vi "Test Sound Measurement.vi"() -> ()   [LabVIEW 2013]
doc: "This VI is used for testing dynamic pressure measurement acquisition with our dynamic pressure sensors and analog input card."
uses:
  <vilib>/DAQmx/read.llb/DAQmx Read (Analog 1D Wfm NChan NSamp).vi
  <vilib>/measure/maspectr.llb/FFT Power Spectrum and PSD for N Chan.vi
  <vilib>/DAQmx/miscellaneous.llb/DAQmx Fill In Error Info.vi
  <vilib>/measure/NI_MAPro.lvlib
panel:
  out "Dynamic Pressure":cluster{"f0":dbl, "df":dbl, "magnitude":dbl[]}[](graph)
  in  "Stop Button":bool
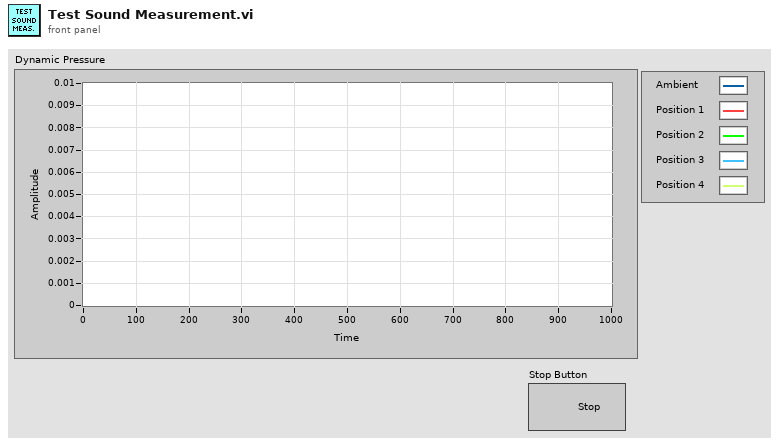
[diagram p1: front panel]
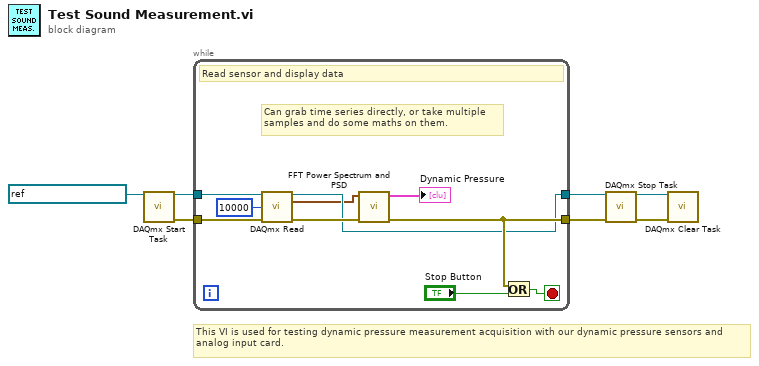
[diagram p0: block diagram]
diagram:
  # "This VI is used for testing dynamic pressure measurement acquisition with our dynamic pressure sensors and analog input card."
  n1 = call <vilib>:"DAQmx Start Task.vi"("task/channels in"=refnum<k21> "DynP_all_S6AI0-4") -> ("task out"=w6:refnum<k21>, "error out"=w7:errorcluster)  [unwired: 13 in]
  n2 = while {
    tunnel: w7 -> [w17]
    tunnel: w6 -> [w16]
    tunnel: [w11] -> w5
    tunnel: [w10] -> w3
    stop <- w15 stop-if-true
    # "Can grab time series directly, or take multiple\nsamples and do some maths on them."
    # "Read sensor and display data"
    n3 = call-poly <vilib>:"DAQmx Read.vi"("task/channels in"=w16, "number of samples per channel"=10000, "error in"=w17) -> ("task out"=w10:refnum<k21>, "data"=w9:waveform(dbl)[], "error out"=w12:errorcluster)  [unwired: 10 in]
    n4 = call-poly <vilib>:"FFT Power Spectrum and PSD.vi"("error in (no error)"=w12, "time signals"=w9) -> ("error out"=w11:errorcluster, "Power Spectrum / PSD"=→"Dynamic Pressure":cluster{"f0":dbl, "df":dbl, "magnitude":dbl[]}[])  [unwired: 6 in, 2 out]
    n5 = Or(x=w11, y="Stop Button") -> (x .or. y?=w15:bool)
  }
  n6 = call <vilib>:"DAQmx Stop Task.vi"("task/channels in"=w3, "error in"=w5) -> ("task out"=w2:refnum<k21>, "error out"=w4:errorcluster)  [unwired: 12 in]
  n7 = call <vilib>:"DAQmx Clear Task.vi"("task in"=w2, "error in"=w4) -> ()  [unwired: 13 in, 1 out]
